vi "Run TS.vi"(8 "error in":errorcluster, 11 "Test Stand in":refnum<class "Generic Test Stand.lvclass">) -> (0 "error out":errorcluster, 3 "Test Stand out":refnum<class "Generic Test Stand.lvclass">)   [LabVIEW 2019, in "Generic Test Stand.lvclass"]
uses:
  Generic Test Stand.lvclass
  TS Panel Method.ctl
  Generic Test Stand.lvclass/Generic Test Stand.ctl
  DAC/DAC.lvclass
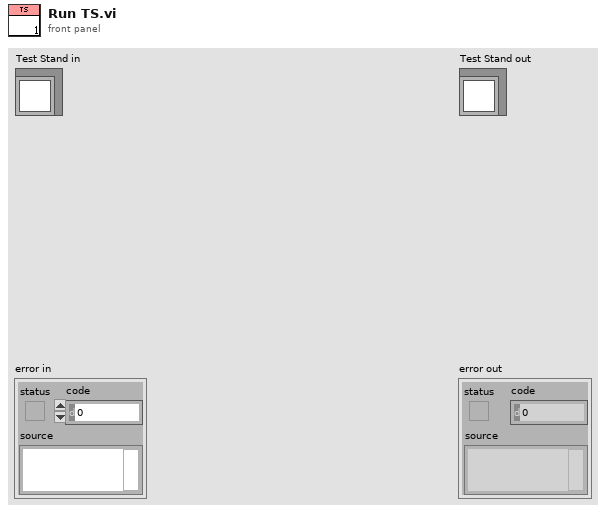
[diagram p1: front panel]
types:
  T1 = typedef "Generic Test Stand.lvclass/TS Panel Method.ctl" = enum16{"Send to Panel", "Receive from Panel", "Update Panel View"}
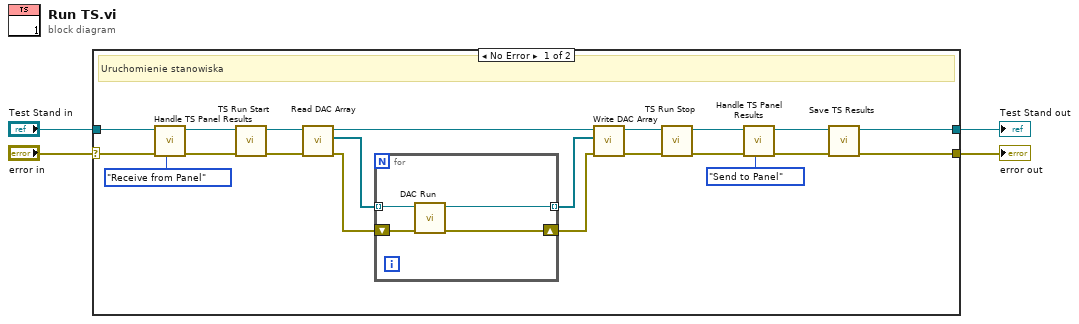
[diagram p0: block diagram]
diagram:
  n1 = case shown="No Error" "error in" {
    selector: "error in" -> [w11 w31]
    tunnel: "Test Stand in" -> [w12 w30]
    tunnel: [w6 w30] -> w3
    tunnel: [w5 w31] -> w1
    frame No Error {
      # "Uruchomienie stanowiska"
      n2 = call-dynamic "Handle TS Panel Results.vi"("Method"=TS_Panel_Method."Receive from Panel", "error in"=w11, "Test Stand in"=w12) -> ("error out"=w17:errorcluster, "Test Stand out"=w19:refnum<class "Generic Test Stand.lvclass">)  [unwired: 7 in]
      n3 = call-dynamic "TS Run Start.vi"("error in (no error)"=w17, "Test Stand in"=w19) -> ("error out"=w8:errorcluster, "Test Stand out"=w18:refnum<class "Generic Test Stand.lvclass">)  [unwired: 8 in]
      n4 = call "Read DAC Array.vi"("error in (no error)"=w8, "Generic Test Stand in"=w18) -> ("error out"=w7:errorcluster, "DAC Array"=w25:refnum<class "DAC.lvclass">[], "Generic Test Stand out"=w24:refnum<class "Generic Test Stand.lvclass">)  [unwired: 7 in]
      n5 = for {
        tunnel: w25 -> [w29] mode=indexing
        shift-right: [w26] -> w22
        shift-left: w7 -> [w28]
        tunnel: [w27] -> w23 mode=indexing
        n6 = call-dynamic "DAC Run.vi"("error in (no error)"=w28, "DAC in"=w29) -> ("error out"=w26:errorcluster, "DAC out"=w27:refnum<class "DAC.lvclass">)  [unwired: 8 in]
      }
      n7 = call "Write DAC Array.vi"("error in (no error)"=w22, "DAC Array"=w23, "Generic Test Stand in"=w24) -> ("error out"=w15:errorcluster, "Generic Test Stand out"=w16:refnum<class "Generic Test Stand.lvclass">)  [unwired: 7 in]
      n8 = call-dynamic "TS Run Stop.vi"("error in (no error)"=w15, "Test Stand in"=w16) -> ("error out"=w13:errorcluster, "Test Stand out"=w14:refnum<class "Generic Test Stand.lvclass">)  [unwired: 8 in]
      n9 = call-dynamic "Handle TS Panel Results.vi"("Method"=TS_Panel_Method."Send to Panel", "error in"=w13, "Test Stand in"=w14) -> ("error out"=w9:errorcluster, "Test Stand out"=w10:refnum<class "Generic Test Stand.lvclass">)  [unwired: 7 in]
      n10 = call-dynamic "Save TS Results.vi"("error in"=w9, "Test Stand in"=w10) -> ("error out"=w5:errorcluster, "Test Stand out"=w6:refnum<class "Generic Test Stand.lvclass">)  [unwired: 8 in]
    }
    frame Error {
    }
  }
  "error out" <- w1
  "Test Stand out" <- w3
